vi "test.timestamp_json.vi"() -> ()   [LabVIEW 2020]
uses:
  timestampMetadata/timestampMetadata.lvclass
  ts.iso8601/ts.iso8601.lvclass
  ts.epochOfTimeUnit/ts.epochOfTimeUnit.lvclass
  C:/code/labview-client/lv_src/ts.absoloute type/ts.absoloute type.lvclass
  ts.absoloute/ts.absoloute.lvclass
  C:/code/labview-client/lv_src/timestampType/timestampType.lvclass
  ts.epochOfTimeUnit/ts.epochOfTimeUnit.lvclass/ts.epochOfTimeUnit.ctl
  ts.absoloute/ts.absoloute.lvclass/ts.absoloute.ctl
  timestampMetadata/timestampMetadata.lvclass/timestampMetadata.ctl
  2c29344c-3fab-4f2a-8242-b385841e3bbd.vi
  ts.epochOfTimeUnit/timeUnit.set.vi
  ts.absoloute/absolute.set.vi
  timestampMetadata/seriesName.set.vi
  timestampMetadata/timestampType.set.vi
  <vilib>/JDP Science/JSONtext/Variant to JSON Text.vi
  <vilib>/JDP Science/JSONtext/LVClass Serializer/JSONtext LVClass Serializer.lvclass
  ts.relative/ts.relative.lvclass
  <vilib>/JDP Science/JSONtext/JSONtext.lvlib
panel:
  out "x = y?":bool
  in  "timestampMetadata":T1
  out "<JSON>":string
  out "error out":errorcluster
  out "json":string
  # "\"timestampMetadata\":{\n\"seriesName\":\"nameValue\"\n\n}"
  # "{\n  \"seriesName\":\"tom\",\n  \"timestampType\":{\n    \"type\":\"absolute\",\n    \"absolute\":{\"type\":\"iso8601\"}\n  }\n}"
  # "{\"seriesName\":\"THISISTHESERIESNAME\",\"timestampType\":{\"type\":\"absolute\",\"absolute\":{\"type\":\"iso8601\"}}}"
  # "{\"seriesName\":\"THISISTHESERIESNAME\",\"timestampType\":{\"type\":absolute,\"absolute\":{\"iso8601\":{\"type\":\"iso8601\"}}}}\n{\"seriesName\":\"THISISTHESERIESNAME\",\"timestampType\":{\"absolute\":{\"type\":\"absolute\",\"absolute\":{\"iso8601\":{\"type\":\"iso8601\"}}}}}"
  # "{\"seriesName\":\"THISISTHESERIESNAME\",\"timestampType\":{\"absolute\":{\"type\":\"absolute\",\"absolute\":{\"iso8601\":{\"type\":\"iso8601\"}}}}}"
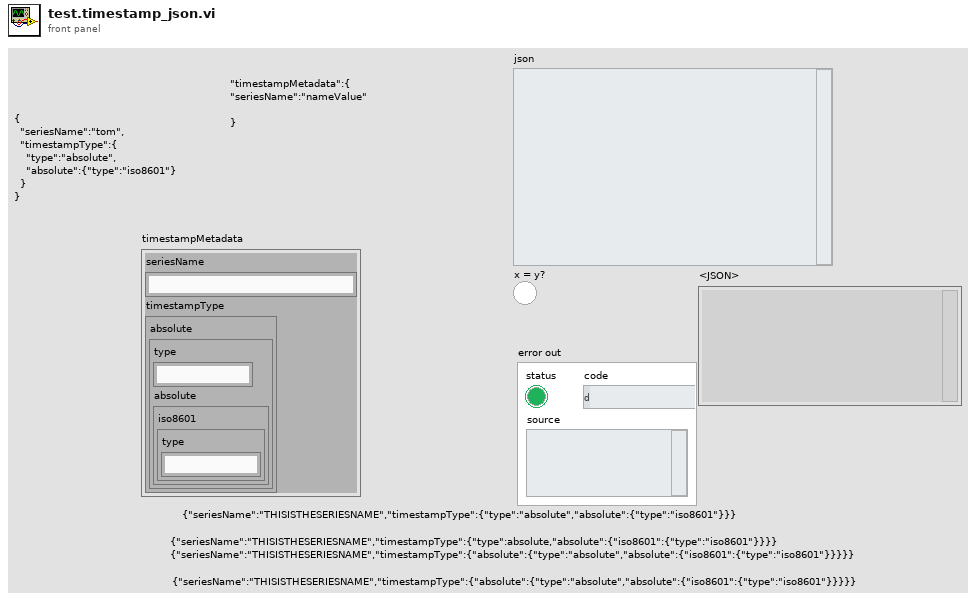
[diagram p1: front panel]
types:
  T1 = cluster{"seriesName":string, "timestampType":cluster{"absolute":cluster{"type":string, "absolute":cluster{"iso8601":cluster{"type":string}}}}}
  T2 = enum16{"DAYS", "HOURS", "MINUTES", "SECONDS", "MILLISECONDS", "MICROSECONDS", "NANOSECONDS", "PICOSECONDS"}
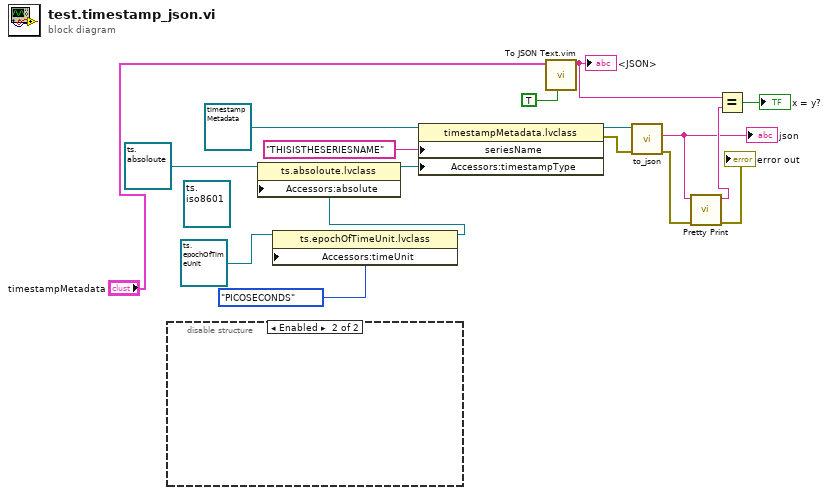
[diagram p0: block diagram]
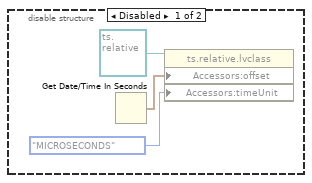
[diagram p2: hidden frame]
diagram:
  (unwired) refnum<class "ts.iso8601.lvclass"> refnum ("ts.iso8601.lvclass")
  n1 = disable-structure shown="Enabled" {
    frame Disabled {
      n2 = Get Date/Time In Seconds() -> (seconds since 1Jan1904=w18:timestamp)
      n3 = property class="ts.relative.lvclass"(reference=refnum<class "ts.relative.lvclass"> refnum ("ts.relative.lvclass"), "Accessors:offset"=w18, "Accessors:timeUnit"=T2."MICROSECONDS" ("timeUnit")) -> ()  [unwired: 1 in, 2 out]
    }
    frame Enabled {
    }
  }
  n4 = property class="ts.epochOfTimeUnit.lvclass"(reference=refnum<class "ts.epochOfTimeUnit.lvclass"> refnum ("ts.epochOfTimeUnit.lvclass"), "Accessors:timeUnit"=T2."PICOSECONDS" ("timeUnit")) -> (reference out=w2:refnum<class "ts.epochOfTimeUnit.lvclass">)  [unwired: 1 in, 1 out]
  n5 = property class="ts.absoloute.lvclass"(reference=refnum<class "ts.absoloute.lvclass"> refnum ("ts.absoloute.lvclass"), "Accessors:absolute"=w2) -> (reference out=w12:refnum<class "ts.absoloute.lvclass">)  [unwired: 1 in, 1 out]
  n6 = property class="timestampMetadata.lvclass"(reference=refnum<class "timestampMetadata.lvclass"> refnum ("timestampMetadata.lvclass"), "seriesName"="THISISTHESERIESNAME", "Accessors:timestampType"=w12) -> (reference out=w15:refnum<class "timestampMetadata.lvclass">, error out=w14:errorcluster)  [unwired: 1 in]
  n7 = call "To JSON Text.vim"("Pretty Print?"=TRUE, "Anything"="timestampMetadata") -> ("<JSON>"=w10:string)  [unwired: 8 in, 1 out]
  "<JSON>" <- w10
  n8 = call-dynamic "to_json.vi"("error in"=w14, "timestampMetadata in"=w15) -> ("error out"=w8:errorcluster, "json"=w4:string)  [unwired: 6 in, 2 out]
  "json" <- w4
  n9 = call <vilib>:"Pretty Print.vi"("error in (no error)"=w8, "JSON"=w4) -> ("error out"=→"error out":errorcluster, "<JSON>"=w6:string)  [unwired: 7 in, 1 out]
  n10 = Equal?(x=w10, y=w6) -> (x = y?=→"x = y?":bool)
